vi "Actor Core.vi"(8 "error in":errorcluster, 11 "SongBrowserActor in":refnum<class "SongBrowserActor.lvclass">) -> (0 "error out":errorcluster, 3 "Actor out":refnum<class "Actor.lvclass">)   [LabVIEW 2015, in "SongBrowserActor.lvlib" / "SongBrowserActor.lvclass"]
doc: "(<B>Filename</B>: Actor Framework.lvlib:Actor.lvclass:Actor Core.vi)\n\nReceives messages to the actor, reacts to them, and initiates any error handling that may shut the actor down.\n\nDescendant classes may override this VI to append parallel tasks for the actor to complete while it handles messages. Overrides use the Call Parent Method node."
uses:
  SongBrowserActor.lvclass
  <vilib>/ActorFramework/Actor/Actor.lvclass
  builds/xctls/Song Browser/Song Browser.lvlibp/app/xctls/Song Browser/Song Browser.xctl
  builds/xctls/Artist Browser/Artist Browser.lvlibp/app/xctls/Artist Browser/Artist Browser.xctl
  builds/xctls/Album Browser/Album Browser.lvlibp/app/xctls/Album Browser/Album Browser/Album Browser.xctl
  SongBrowserActor.lvclass/SongBrowserActor.ctl
  <vilib>/ActorFramework/Actor/Actor.lvclass/Actor.ctl
  <vilib>/ActorFramework/Message Enqueuer/Message Enqueuer.lvclass/Message Enqueuer.ctl
  <vilib>/ActorFramework/Message Enqueuer/Init from Existing Queue.vi
  <vilib>/ActorFramework/Message Enqueuer/Enqueue.vi
  <vilib>/ActorFramework/Message Priority Queue/Priority Enqueue.vi
  <vilib>/ActorFramework/Message Enqueuer/Message Enqueuer.lvclass
  <vilib>/ActorFramework/Stop Msg/Stop Msg.lvclass
  MusicManagerActor/MusicManagerActor Messages/View Song Library Request by Artist Msg/View Song Library Request by Artist Msg.lvclass
  MusicManagerActor/MusicManagerActor Messages/View Song Library Request by Album Msg/View Song Library Request by Album Msg.lvclass
  MusicManagerActor/MusicManagerActor Messages/Enqueue Song Requested by UID Msg/Enqueue Song Requested by UID Msg.lvclass
panel:
  in  "UI Tabs":enum32{"Main", "Debug"}(tab)
  out "Number Of Elements":string
  out "List Name":string
  in  "Array Panel":enum32{"Songs", "Artists", "Albums"}(tab)
  in  "Song Browser":T1[](xcontrol)
  in  "Artist Browser":T4[](xcontrol)
  in  "Album Browser":T6[](xcontrol)
  # "Make the menu items x controls to change text when hovers over"
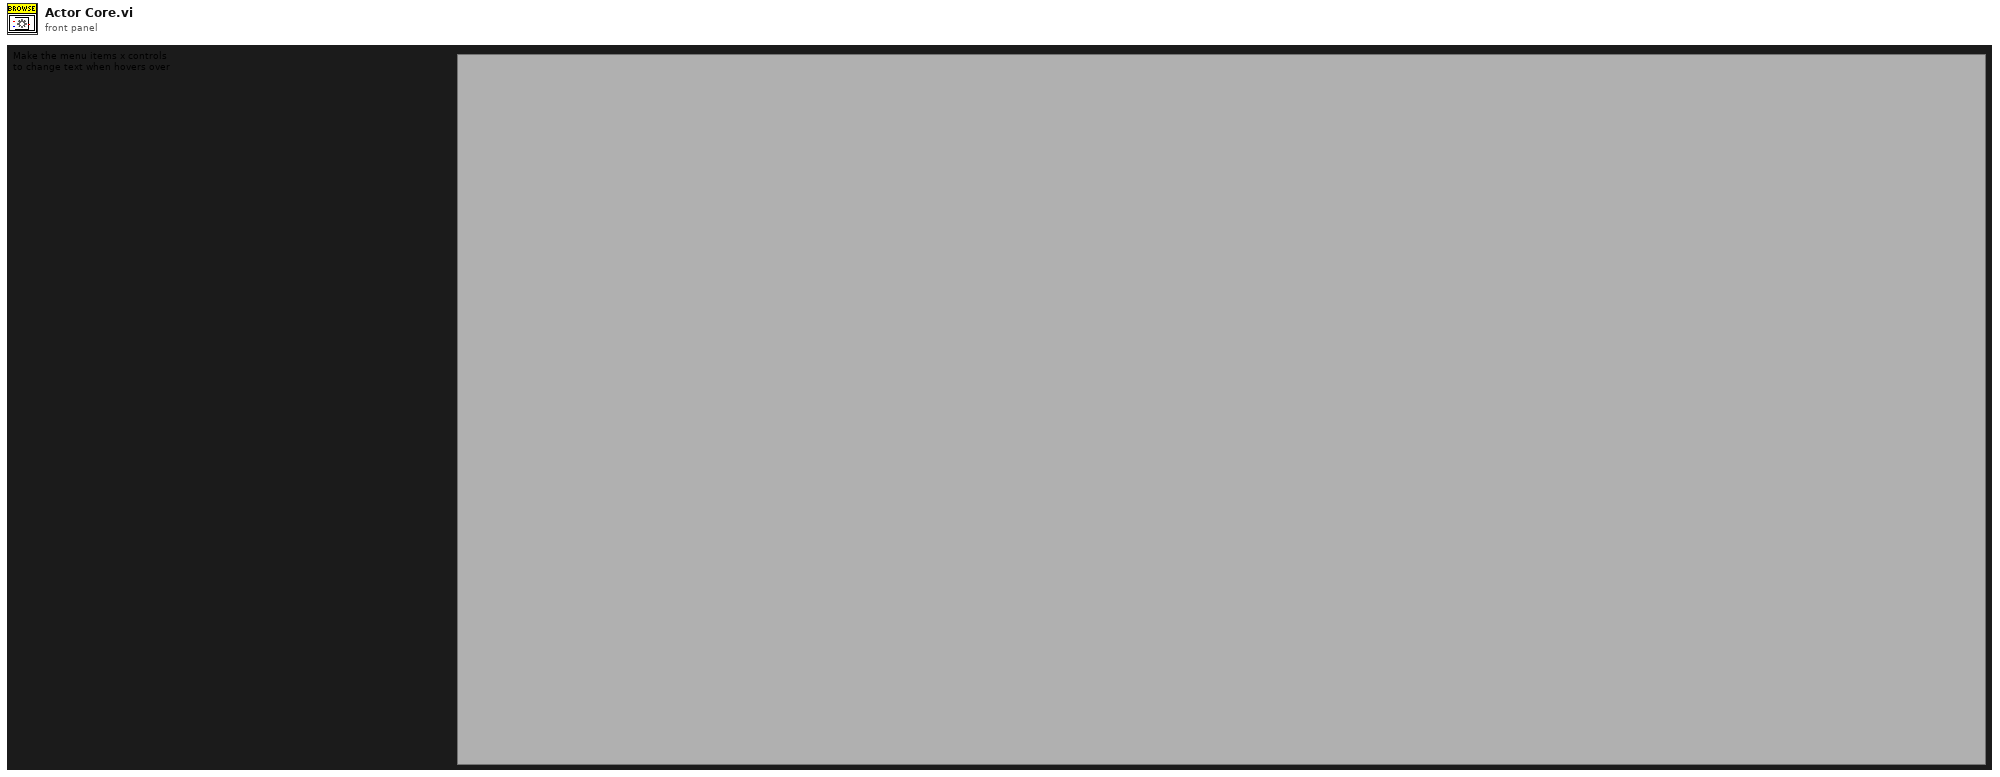
[diagram p1: front panel]
types:
  T1 = typedef "Song Browser.lvlibp/Queue Song Display.ctl" = cluster{"Song Name":string, "Artist":string, "Album":string, "Duration (s)":T2, "UID":string, "Dequeue":T3}
  T2 = typedef "Song Browser.lvlibp/Song.lvclass/Song Duration.ctl" = timestamp
  T3 = typedef "Song Browser.lvlibp/Dequeue Control.ctl" = bool
  T4 = typedef "Artist Browser.lvlibp/Music Library Element Display.ctl" = cluster{"Name":string, "Details":string, "Duration (s)":T5, "Click":bool}
  T5 = typedef "Artist Browser.lvlibp/Song.lvclass/Song Duration.ctl" = timestamp
  T6 = typedef "Album Browser.lvlibp/Music Library Element Display.ctl" = cluster{"Name":string, "Details":string, "Duration (s)":T7, "Click":bool}
  T7 = typedef "Album Browser.lvlibp/Song.lvclass/Song Duration.ctl" = timestamp
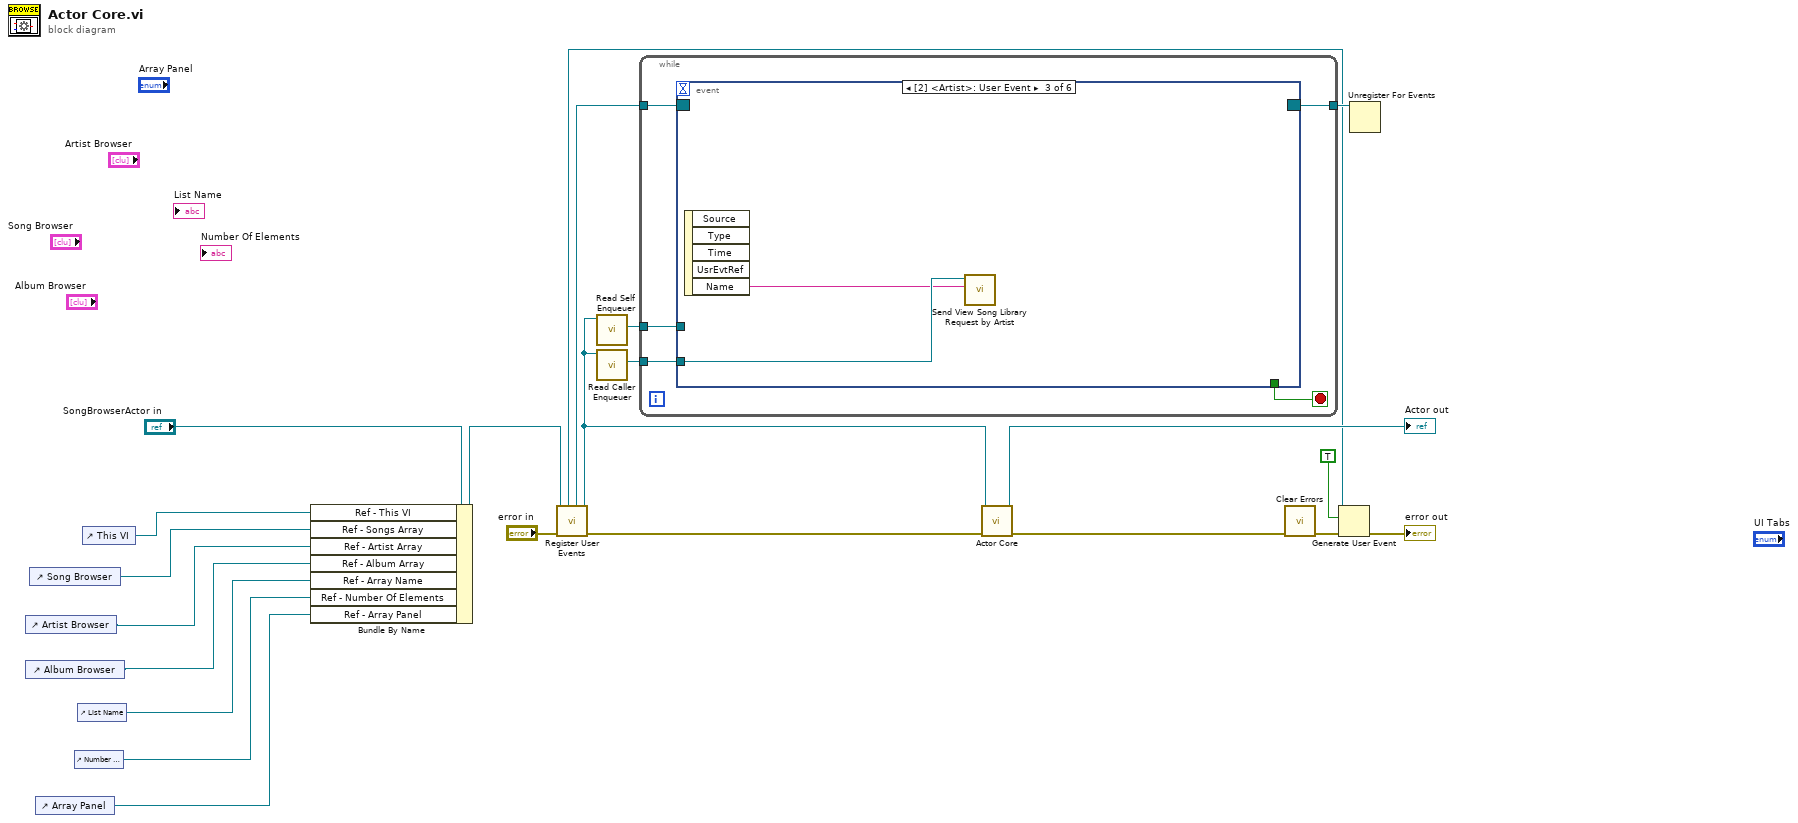
[diagram p0: block diagram]
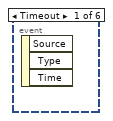
[diagram p2: hidden frame]
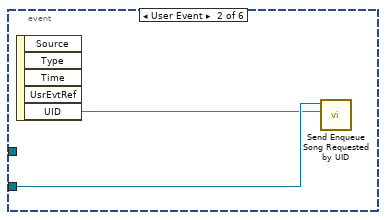
[diagram p3: hidden frame]
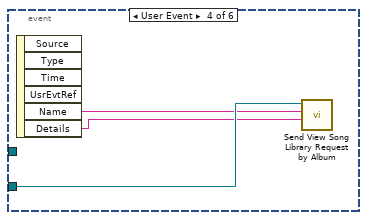
[diagram p4: hidden frame]
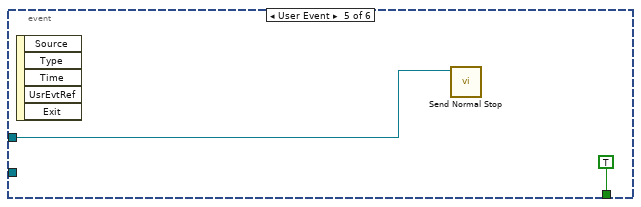
[diagram p5: hidden frame]
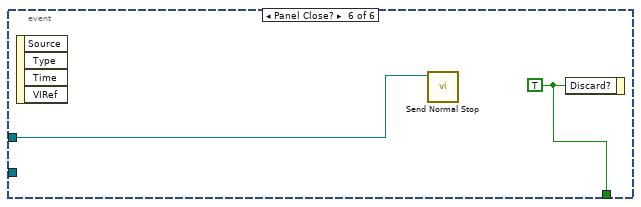
[diagram p6: hidden frame]
diagram:
  n1 = control-ref of="Artist Browser"() -> (w8:refnum<vi>)
  n2 = control-ref of="Album Browser"() -> (w7:refnum<vi>)
  n3 = control-ref of="Song Browser"() -> (w9:refnum<vi>)
  n4 = control-ref of="Array Panel"() -> (w10:refnum<vi>)
  n5 = control-ref of="Number Of Elements"() -> (w11:refnum<vi>)
  n6 = control-ref of="List Name"() -> (w12:refnum<vi>)
  n7 = control-ref of="This VI"() -> (w13:refnum<vi>)
  n8 = Bundle By Name(cluster="SongBrowserActor in", "Ref - This VI"=w13, "Ref - Songs Array"=w9, "Ref - Artist Array"=w8, "Ref - Album Array"=w7, "Ref - Array Name"=w12, "Ref - Number Of Elements"=w11, "Ref - Array Panel"=w10) -> (w5:refnum<class "SongBrowserActor.lvclass">)
  n9 = call "Register User Events.vi"("error in (no error)"="error in", "SongBrowserActor in"=w5) -> ("error out"=w3:errorcluster, "SongBrowserActor out"=w4:refnum<class "SongBrowserActor.lvclass">, "Event Registration Refnum"=w1:refnum<event-registration>, "Exit Event"=w2:refnum<user-event>)  [unwired: 6 in]
  n10 = call <vilib>:"Read Self Enqueuer.vi"("Actor"=w4) -> ("Self Enqueuer"=w18:refnum<class "Message Enqueuer.lvclass">)  [unwired: 10 in]
  n11 = call <vilib>:"Read Caller Enqueuer.vi"("Actor"=w4) -> ("Caller Enqueuer"=w15:refnum<class "Message Enqueuer.lvclass">)  [unwired: 10 in]
  n12 = while {
    tunnel: w1 -> [w27]
    tunnel: [w25] -> w22
    tunnel: w18 -> [w24]
    tunnel: w15 -> [w23]
    stop <- w26 stop-if-true
    n13 = event shown="[2] <Artist>: User Event" {
      selector: w27 -> [_ _ _ _ _ _]
      dyn-events: [_ _ _ _ _ _] -> w25
      timeout: _ -> [_ _ _ _ _ _]
      tunnel: [_ _ _ _ TRUE ("Exit") w38] -> w26
      tunnel: w24 -> [_ _ _ _ w35 w37]
      tunnel: w23 -> [_ w29 w31 w34 _ _]
      event Timeout {
        n14 = event-data() -> ()  [unwired: 1 in, 3 out]
      }
      event User Event {
        n15 = event-data() -> ("UID"=w28:string)  [unwired: 1 in, 4 out]
        n16 = call "Send Enqueue Song Requested by UID.vi"("Song UID"=w28, "Message Enqueuer in"=w29) -> ()  [unwired: 8 in, 2 out]
      }
      event User Event {
        n17 = event-data() -> ("Name"=w30:string)  [unwired: 1 in, 4 out]
        n18 = call "Send View Song Library Request by Artist.vi"("Artist"=w30, "Message Enqueuer in"=w31) -> ()  [unwired: 8 in, 2 out]
      }
      event User Event {
        n19 = event-data() -> ("Name"=w33:string, "Details"=w32:string)  [unwired: 1 in, 4 out]
        n20 = call "Send View Song Library Request by Album.vi"("Artist"=w32, "Album"=w33, "Message Enqueuer in"=w34) -> ()  [unwired: 7 in, 2 out]
      }
      event User Event {
        n21 = event-data() -> ()  [unwired: 1 in, 5 out]
        n22 = call <vilib>:"Send Normal Stop.vi"("Message Enqueuer"=w35) -> ()  [unwired: 10 in, 1 out]
      }
      event Panel Close? {
        w38 = TRUE ("Discard?")
        n23 = event-data() -> ()  [unwired: 1 in, 4 out]
        n24 = call <vilib>:"Send Normal Stop.vi"("Message Enqueuer"=w37) -> ()  [unwired: 10 in, 1 out]
        n25 = event-data("Discard?"=w38) -> ()  [unwired: 1 in, 1 out]
      }
    }
  }
  n26 = call-parent "Actor Core.vi"("error in"=w3, "Actor in"=w4) -> ("error out"=w21:errorcluster, "Actor out"=→"Actor out":refnum<class "Actor.lvclass">)  [unwired: 8 in]
  n27 = call <vilib>:"Clear Errors.vi"("error in (no error)"=w21) -> ("error out"=w19:errorcluster)  [unwired: 5 in, 1 out]
  n28 = Generate User Event(user event=w2, event data cluster=TRUE ("event data"), error in=w19) -> (error out=→"error out":errorcluster)  [unwired: 1 in, 1 out]
  n29 = Unregister For Events(event registration refnum=w22) -> ()  [unwired: 1 in, 1 out]
